vi "Get Level.vi"(6 "Output Channel":T1, 8 "error in (no error)":errorcluster, 11 "Inst.RP100 in":refnum<class "Inst.RP100.lvclass">) -> (0 "error out":errorcluster, 2 "Level (V)":dbl, 3 "Inst.RP100 out":refnum<class "Inst.RP100.lvclass">)   [LabVIEW 2019, in "Inst.RP100.lvlib" / "Inst.RP100.lvclass"]
uses:
  Inst.RP100.lvclass
  Typedefs/Channel--Num.ctl
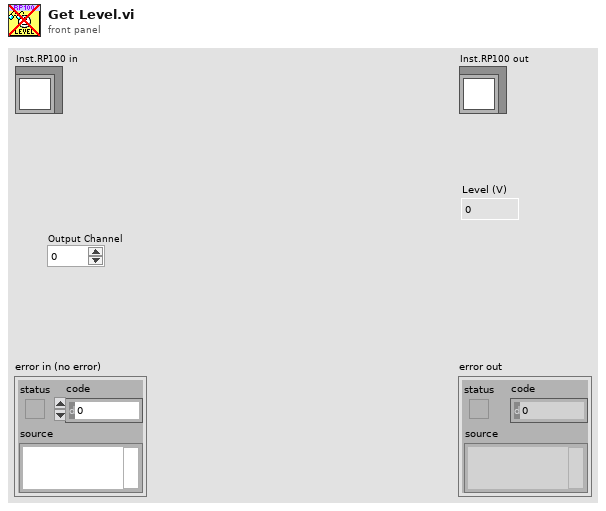
[diagram p1: front panel]
types:
  T1 = typedef "Inst.RP100.lvlib/Inst.RP100.lvclass/Channel--Num.ctl" = i32
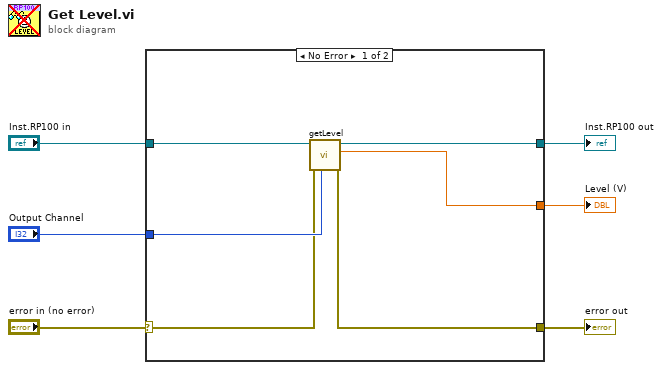
[diagram p0: block diagram]
diagram:
  n1 = case shown="No Error" "error in (no error)" {
    selector: "error in (no error)" -> [w7 w14]
    tunnel: [w8 w14] -> w5
    tunnel: "Inst.RP100 in" -> [w10 w13]
    tunnel: [w9 w13] -> w3
    tunnel: [w12 _] -> w1
    tunnel: "Output Channel" -> [w11 _]
    frame No Error {
      n2 = call-dynamic "getLevel.vi"("Output Channel"=w11, "error in (no error)"=w7, "Inst.RP100 in"=w10) -> ("error out"=w8:errorcluster, "Level (V)"=w12:dbl, "Inst.RP100 out"=w9:refnum<class "Inst.RP100.lvclass">)  [unwired: 6 in]
    }
    frame Error {
    }
  }
  "error out" <- w5
  "Inst.RP100 out" <- w3
  "Level (V)" <- w1
